vi "LTS_Channel Switching.vi"() -> ()   [LabVIEW 2022 SP3]
uses:
  <instrlib>/Keithley DMM6500 DAQ6500 Series/Keithley DMM6500 DAQ6500 Series.lvlib
panel:
  out "String Array of Selected Channels":string[](array[string])
  out "Index Array of Selected Channels":i32[](array[numeric])
  in  "Channels":i32[](listbox)
  out "String Array of Selected items":string[](array[string])
  out "Array of Selected Items":i32[](array[numeric])
  in  "Channels":i32[](listbox)
  in  "Interface":string(combo)
  out "error out":errorcluster
  out "VISA resource name out":refnum<visa-resource-name>
  in  "error in (no error)":errorcluster
  in  "VISA resource name":refnum<visa-resource-name>
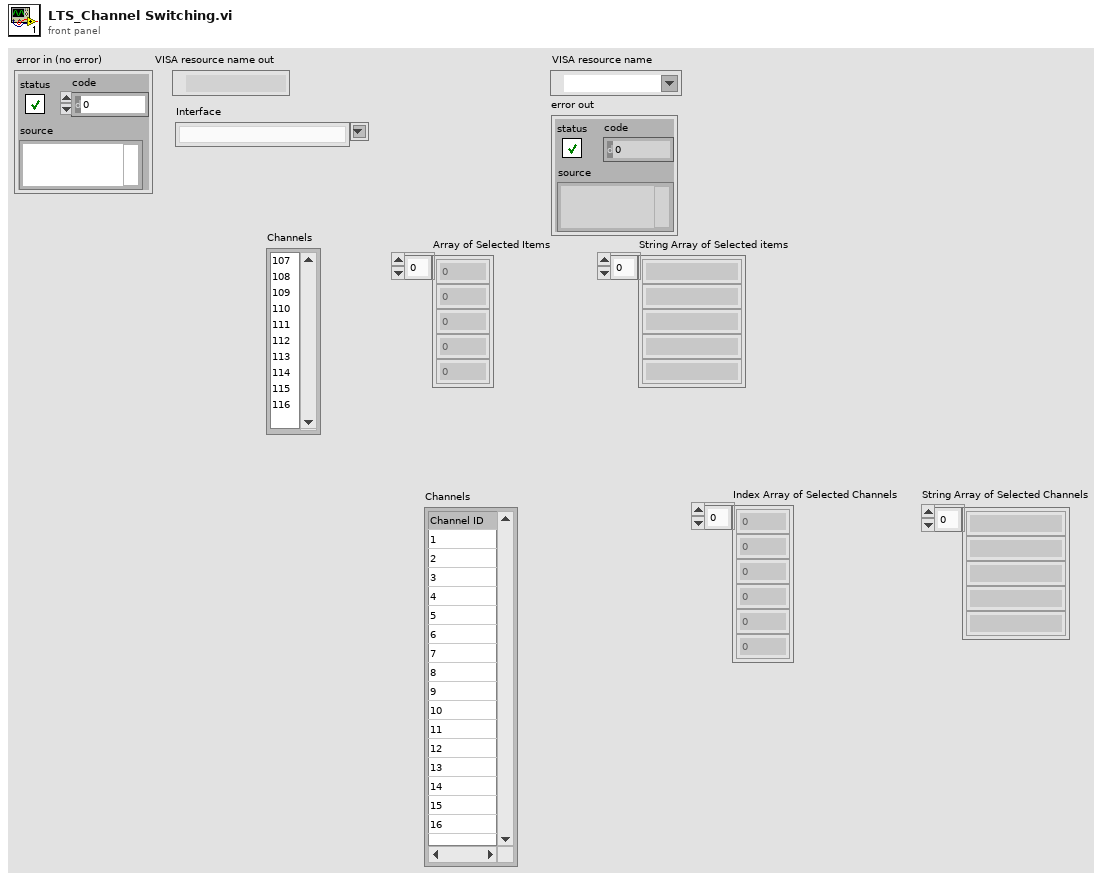
[diagram p1: front panel]
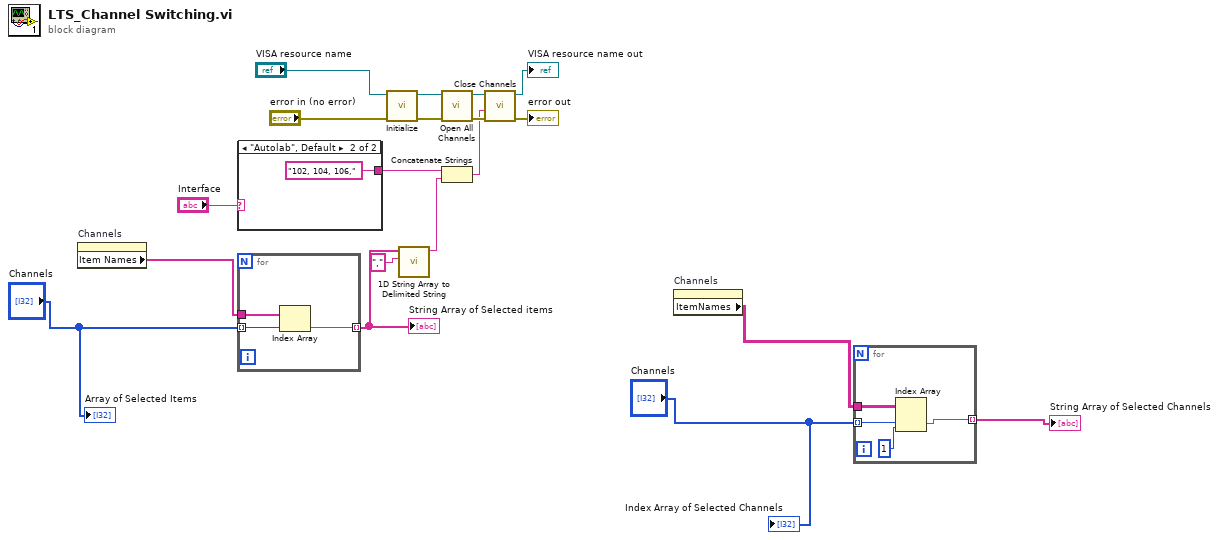
[diagram p0: block diagram]
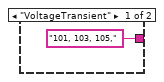
[diagram p2: hidden frame]
diagram:
  n1 = property on="Channels" class="LstBox (strict)"() -> ("Item Names"=w10:string[])  [unwired: 2 in, 2 out]
  n2 = case shown="\"Autolab\", Default" "Interface" {
    tunnel: ["101, 103, 105," "102, 104, 106,"] -> w9
    frame "VoltageTransient" {
    }
    frame "Autolab", Default {
    }
  }
  n3 = for {
    tunnel: "Channels" -> [w23] mode=indexing
    tunnel: w10 -> [w24]
    tunnel: [w22] -> w4 mode=indexing
    n4 = Index Array(array=w24, index=w23) -> (element=w22:string)
  }
  "String Array of Selected items" <- w4
  n5 = call <instrlib>:"Initialize.vi"("error in (no error)"="error in (no error)", "VISA resource name"="VISA resource name") -> ("error out"=w17:errorcluster, "VISA resource name out"=w15:refnum<visa-resource-name>)  [unwired: 8 in]
  n6 = call <vilib>:"1D String Array to Delimited String.vi"("delimiter"=",", "string array"=w4) -> ("delimited string"=w6:string)  [unwired: 9 in]
  n7 = call <instrlib>:"Open All Channels.vi"("error in (no error)"=w17, "VISA resource name"=w15) -> ("error out"=w16:errorcluster, "VISA resource name out"=w14:refnum<visa-resource-name>)  [unwired: 8 in]
  n8 = Concatenate Strings(w9, w6) -> (w8:string)
  n9 = call <instrlib>:"Close Channels.vi"("error in (no error)"=w16, "Channel List(\"\")"=w8, "VISA resource name"=w14) -> ("error out"=→"error out":errorcluster, "VISA resource name out"=→"VISA resource name out":refnum<visa-resource-name>)  [unwired: 7 in]
  n10 = property on="Channels" class="MCListbox (strict)"() -> ("ItemNames"=w3:string[][])  [unwired: 2 in, 2 out]
  n11 = for {
    tunnel: w3 -> [w28]
    tunnel: "Channels" -> [w26] mode=indexing
    tunnel: [w27] -> w1 mode=indexing
    n12 = Index Array(array=w28, index (row)=w26, index (col)=1 ("disabled index (col)")) -> (element=w27:string)
  }
  "String Array of Selected Channels" <- w1
  "Array of Selected Items" <- "Channels"
  "Index Array of Selected Channels" <- "Channels"
